vi "Ignore if in LabVIEW Directory.vi"(8 "error in":errorcluster, 11 "Dep Names and Paths":T1) -> (0 "error out":errorcluster, 3 "Filtered Dep Names and Paths":T1)   [LabVIEW 2018, in "Name and Dependency Processing.lvlib"]
uses:
  Name and Dependency Processing.lvlib
  Dep Names and Paths.ctl
  <vilib>/regexp/Match Regular Expression.xnode
  Path and string processing/Path and String Processing.lvlib
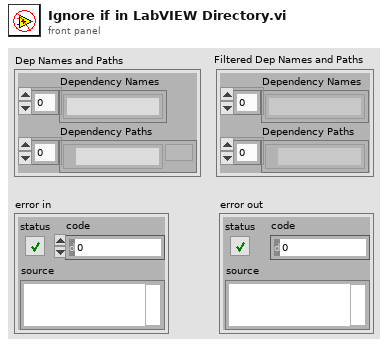
[diagram p1: front panel]
types:
  T1 = typedef "Name and Dependency Processing.lvlib/Dep Names and Paths.ctl" = cluster{"Dependency Names":string[], "Dependency Paths":path[]}
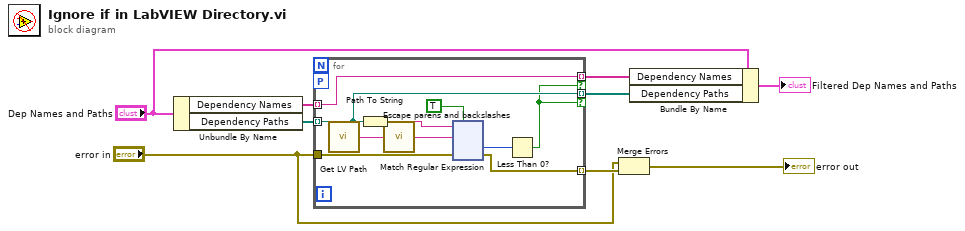
[diagram p0: block diagram]
diagram:
  n1 = Unbundle By Name("Dep Names and Paths") -> ("Dependency Names"=w9:string[], "Dependency Paths"=w8:path[])
  n2 = for {
    tunnel: w8 -> [w11] mode=indexing
    tunnel: w9 -> [w17] mode=indexing
    tunnel: [w17] -> w4 mode=indexing if=w10
    workers-P: _ -> [_]
    tunnel: "error in" -> [w13]
    tunnel: [w12] -> w7 mode=indexing
    tunnel: [w11] -> w2 mode=indexing if=w10
    n3 = call "Get LV Path.vi"() -> ("String"=w16:string)
    n4 = Path To String(path=w11) -> (string=w14:string)
    n5 = call "Escape parens and backslashes.vi"("Input String"=w16) -> ("Escaped String"=w15:string)  [unwired: 14 in]
    n6 = xnode "Match Regular Expression"("input string"=w14, "regular expression"=w15, "error in"=w13, "ignore case? (F)"=TRUE) -> ("offset past match"=w19:i32, "error out"=w12:errorcluster)  [unwired: 2 in, 3 out]
    n7 = Less Than 0?(x=w19) -> (x < 0?=w10:bool)
  }
  n8 = Merge Errors("error in", w7) -> (→"error out":errorcluster)
  n9 = Bundle By Name(cluster="Dep Names and Paths", "Dependency Names"=w4, "Dependency Paths"=w2) -> (→"Filtered Dep Names and Paths":T1)
